vi "duty_cycle_control.vi"(8 "error in (no error)":errorcluster, 9 "Duty Cycle (%)":dbl(slide) scale=0.0..100.0, 10 "Pin":u8 max=7 step=1, 11 "VISA resource name":refnum<visa-resource-name>) -> (0 "error out":errorcluster, 3 "VISA resource name out":refnum<visa-resource-name>)   [LabVIEW 2023]
uses:
  pico_scpi_labtool_labview_driver/scpi_driver/usbtmc_scpi_labtool.lvlib
panel:
  # "Pin 0 - GP16\nPin 1 - GP17\nPin 2 - GP18"
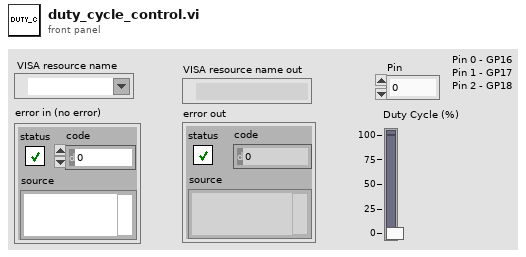
[diagram p1: front panel]
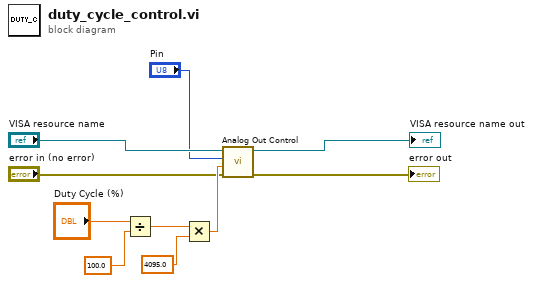
[diagram p0: block diagram]
diagram:
  n1 = Divide(x="Duty Cycle (%)", y=100.0) -> (x/y=w5:dbl)
  n2 = Multiply(x=w5, y=4095.0) -> (x*y=w4:dbl)
  n3 = call "Analog Out Control.vi"("VISA resource name"="VISA resource name", "Pin"="Pin", "duty cycle"=w4, "error in (no error)"="error in (no error)") -> ("VISA resource name out"=→"VISA resource name out":refnum<visa-resource-name>, "error out"=→"error out":errorcluster)  [unwired: 5 in]
